vi "Assign Error.vi"(8 "error in (no error)":errorcluster, 11 "Array":bool[](array[boolean])) -> (0 "error out":errorcluster)   [LabVIEW 2026, in "Settings.lvlib"]
uses:
  Settings.lvlib
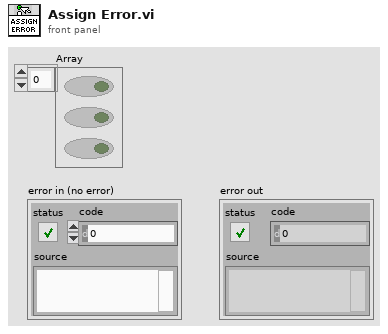
[diagram p1: front panel]
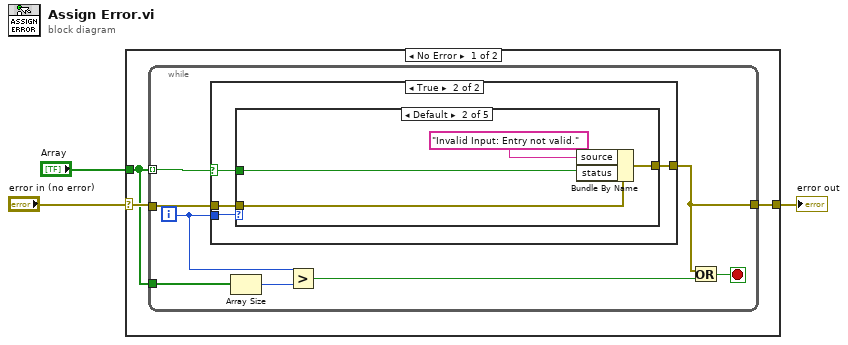
[diagram p0: block diagram]
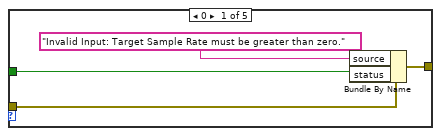
[diagram p3: hidden frame]
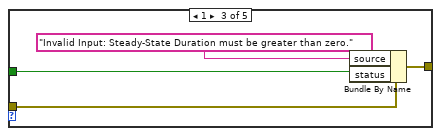
[diagram p4: hidden frame]
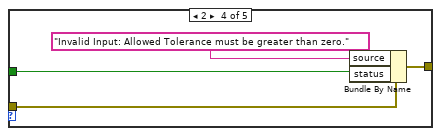
[diagram p5: hidden frame]
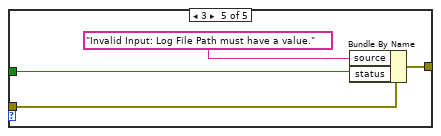
[diagram p6: hidden frame]
diagram:
  n1 = case shown="No Error" "error in (no error)" {
    selector: "error in (no error)" -> [w5 w40]
    tunnel: [w6 w40] -> w3
    tunnel: "Array" -> [w4 _]
    frame No Error {
      n2 = while {
        tunnel: w4 -> [w13] mode=indexing
        tunnel: w5 -> [w14]
        tunnel: [w8] -> w6
        tunnel: w4 -> [w12]
        i -> [w10]
        stop <- w7 stop-if-true
        n3 = case shown="True" w13 {
          selector: w13 -> [_ w17]
          tunnel: w10 -> [_ w19]
          tunnel: w14 -> [w15 w18]
          tunnel: [w15 w16] -> w8
          frame False {
          }
          frame True {
            n4 = case shown="Default" w19 {
              tunnel: w18 -> [w23 w27 w31 w35 w39]
              tunnel: w17 -> [w22 w26 w30 w34 w38]
              tunnel: [w21 w25 w29 w33 w37] -> w16
              frame 0 {
                n5 = Bundle By Name(cluster=w23, "source"="Invalid Input: Target Sample Rate must be greater than zero.", "status"=w22) -> (w21:errorcluster)
              }
              frame Default {
                n6 = Bundle By Name(cluster=w27, "source"="Invalid Input: Entry not valid.", "status"=w26) -> (w25:errorcluster)
              }
              frame 1 {
                n7 = Bundle By Name(cluster=w31, "source"="Invalid Input: Steady-State Duration must be greater than zero.", "status"=w30) -> (w29:errorcluster)
              }
              frame 2 {
                n8 = Bundle By Name(cluster=w35, "source"="Invalid Input: Allowed Tolerance must be greater than zero.", "status"=w34) -> (w33:errorcluster)
              }
              frame 3 {
                n9 = Bundle By Name(cluster=w39, "source"="Invalid Input: Log File Path must have a value.", "status"=w38) -> (w37:errorcluster)
              }
            }
          }
        }
        n10 = Array Size(array=w12) -> (size(s)=w11:i32)
        n11 = Greater?(x=w10, y=w11) -> (0:w9:bool)
        n12 = Or(x=w8, y=w9) -> (x .or. y?=w7:bool)
      }
    }
    frame Error {
    }
  }
  "error out" <- w3
